vi "TimedTrigger.vi"(8 "error in (no error)":errorcluster, 10 "Time after next UTC Second":T1={"TriggerName"="", "Time after next UTC Second"=0.0, "Trigger Duration"=0.1}, 11 "NiPxi6683H in":refnum<class "NiPxi6683H.lvclass">) -> (0 "error out":errorcluster, 3 "NiPxi6683H out":refnum<class "NiPxi6683H.lvclass">)   [LabVIEW 2014, in "SyncPlugins.lvlib" / "NiPxi6683H.lvclass"]
uses:
  NiPxi6683H.lvclass
  SyncPluginBase/Typedefs/clTimedTrigger.ctl
  NiPxi6683H.lvclass/NiPxi6683H.ctl
  NiPxi6682/NiPxi6682.lvclass/NiPxi6682.ctl
  NiPxi6682/Accessors/Read NiSyncHandle.vi
  NiPxi6682/Accessors/Write NiSyncHandle.vi
  Accessors/Write Triggers.vi
  Accessors/Read Triggers.vi
  <vilib>/Utility/error.llb/Error Cluster From Error Code.vi
  <vilib>/ErrorRing/Error Ring.xnode
  SyncPluginBase/SyncPluginBase.lvclass
panel:
  out "Next PPS 2":timestamp
  out "Next PPS":timestamp
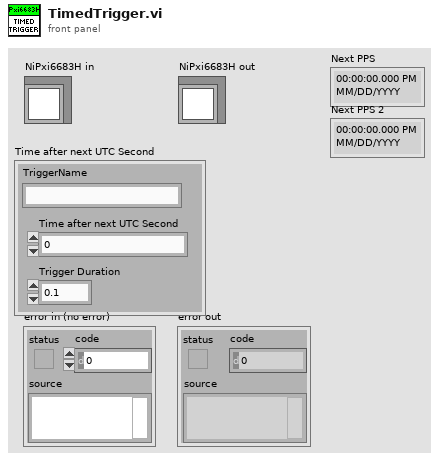
[diagram p1: front panel]
types:
  T1 = typedef "SyncPlugins.lvlib/SyncPluginBase.lvclass/clTimedTrigger.ctl" = cluster{"TriggerName":string, "Time after next UTC Second":dbl, "Trigger Duration":dbl}
  T2 = typedef "SyncPlugins.lvlib/PXI_MultiTrig.lvclass/clTrigger.ctl" = cluster{"Name":string, "DestTerm":string, "SrcTerm":string, "SyncClk":string, "Edge":i32, "Invert?":i32, "Initiated":bool, "Type":string, "TrigTime":bool}
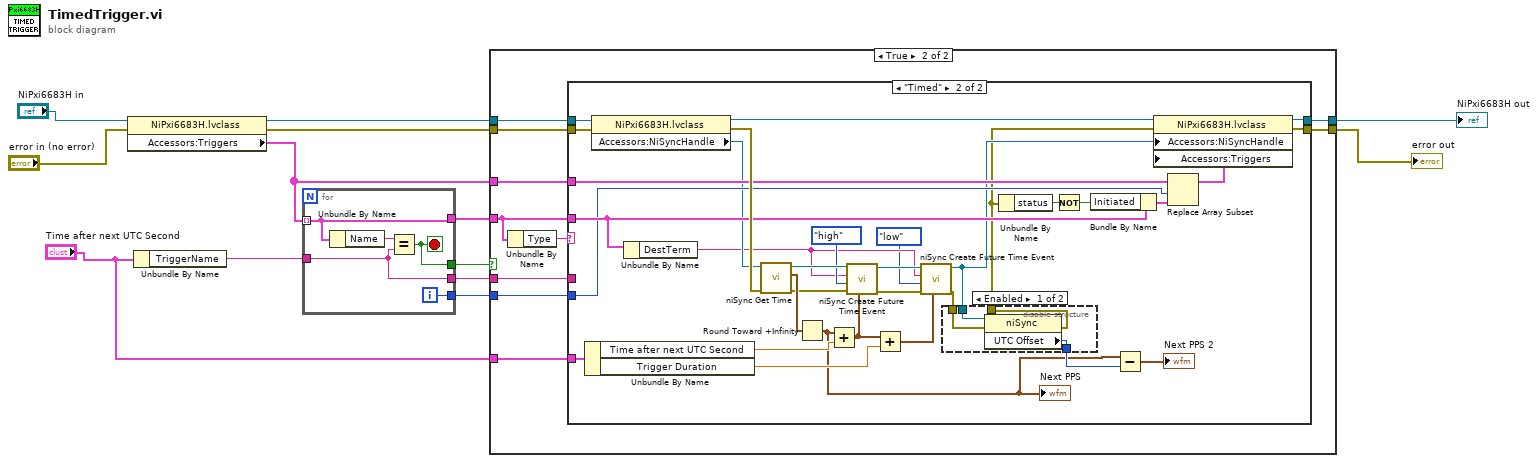
[diagram p0: block diagram]
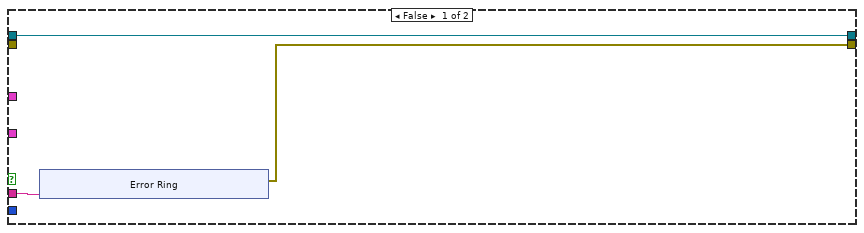
[diagram p2: hidden frame]
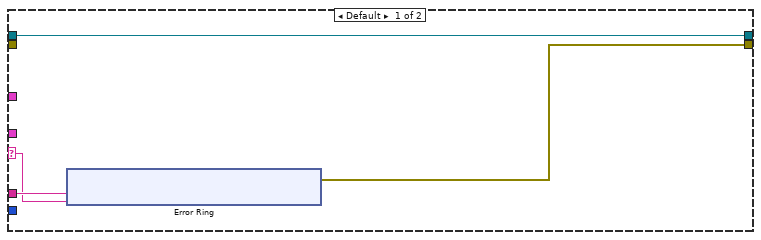
[diagram p3: hidden frame]
diagram:
  n1 = property class="NiPxi6683H.lvclass"(reference="NiPxi6683H in", error in="error in (no error)") -> (reference out=w10:refnum<class "NiPxi6683H.lvclass">, error out=w9:errorcluster, "Accessors:Triggers"=w6:T2[])
  n2 = Unbundle By Name("Time after next UTC Second") -> ("TriggerName"=w13:string)
  n3 = for {
    tunnel: w6 -> [w17] mode=indexing
    tunnel: w13 -> [w15]
    tunnel: [w17] -> w8
    tunnel: [w16] -> w12
    tunnel: [w15] -> w11
    tunnel: [w14] -> w7
    i -> [w14]
    stop <- w16 stop-if-true
    n4 = Unbundle By Name(w17) -> ("Name"=w18:string)
    n5 = Equal?(x=w18, y=w15) -> (x = y?=w16:bool)
  }
  n6 = case shown="True" w12 {
    tunnel: w11 -> [w21 w37]
    tunnel: w10 -> [w20 w32]
    tunnel: w9 -> [_ w30]
    tunnel: [w20 w31] -> w2
    tunnel: [w19 w34] -> w1
    tunnel: w8 -> [_ w33]
    tunnel: w7 -> [_ w36]
    tunnel: w6 -> [_ w35]
    tunnel: "Time after next UTC Second" -> [_ w29]
    frame False {
      n7 = xnode "Error Ring"("parameter 0"=w21) -> ("error out"=w19:errorcluster)
    }
    frame True {
      n8 = Unbundle By Name(w33) -> ("Type"=w38:string)
      n9 = case shown="\"Timed\"" w38 {
        selector: w38 -> [w41 _]
        tunnel: w37 -> [w42 _]
        tunnel: w36 -> [_ w70]
        tunnel: w35 -> [_ w71]
        tunnel: [w40 w76] -> w34
        tunnel: w33 -> [_ w75]
        tunnel: w32 -> [w39 w82]
        tunnel: [w39 w77] -> w31
        tunnel: w30 -> [_ w83]
        tunnel: w29 -> [_ w59]
        frame Default {
          n10 = xnode "Error Ring"("parameter 0"=w42, "parameter 1"=w41) -> ("error out"=w40:errorcluster)
        }
        frame "Timed" {
          n11 = Unbundle By Name(w59) -> ("Time after next UTC Second"=w58:dbl, "Trigger Duration"=w57:dbl)
          n12 = property class="NiPxi6683H.lvclass"(reference=w82, error in=w83) -> (reference out=w78:refnum<class "NiPxi6683H.lvclass">, error out=w81:errorcluster, "Accessors:NiSyncHandle"=w68:refnum<k15>)
          n13 = Unbundle By Name(w75) -> ("DestTerm"=w61:string)
          n14 = call <instrlib>:"niSync Get Time.vi"("error in (no error)"=w81, "instrument handle"=w68) -> ("error out"=w79:errorcluster, "time"=w80:timestamp, "instrument handle out"=w67:refnum<k15>)  [unwired: 5 in]
          n15 = Round Toward +Infinity(x=w80) -> (ceil(x): smallest int >= x=w52:timestamp)
          "Next PPS" <- w52
          n16 = Add(x=w52, y=w58) -> (x+y=w63:timestamp)
          n17 = call <instrlib>:"niSync Create Future Time Event.vi"("time"=w63, "error in (no error)"=w79, "output level"=enum32{"low", "high"}."high", "terminal"=w61, "instrument handle"=w67) -> ("error out"=w65:errorcluster, "instrument handle out"=w64:refnum<k15>)  [unwired: 4 in]
          n18 = Add(x=w63, y=w57) -> (x+y=w62:timestamp)
          n19 = call <instrlib>:"niSync Create Future Time Event.vi"("time"=w62, "error in (no error)"=w65, "output level"=enum32{"low", "high"}."low", "terminal"=w61, "instrument handle"=w64) -> ("error out"=w55:errorcluster, "instrument handle out"=w56:refnum<k15>)  [unwired: 4 in]
          n20 = disable-structure shown="Enabled" {
            disable-tunnel: w56 -> [w87 _]
            disable-tunnel: w55 -> [w86 w88]
            disable-tunnel: [w85 w88] -> w54
            disable-tunnel: [w84 _] -> w53
            frame Enabled {
              n21 = property class="niSync"(reference=w87, error in=w86) -> (error out=w85:errorcluster, "UTC Offset"=w84:i32)  [unwired: 1 out]
            }
            frame Disabled {
            }
          }
          n22 = Unbundle By Name(w54) -> ("status"=w74:bool)
          n23 = Not(x=w74) -> (.not. x?=w73:bool)
          n24 = Bundle By Name(cluster=w75, "Initiated"=w73) -> (w72:T2)
          n25 = Subtract(x=w52, y=w53) -> (x-y=→"Next PPS 2":timestamp)
          n26 = Replace Array Subset(array=w71, new element=w72, index=w70) -> (w69:T2[])
          n27 = property class="NiPxi6683H.lvclass"(reference=w78, error in=w54, "Accessors:NiSyncHandle"=w56, "Accessors:Triggers"=w69) -> (reference out=w77:refnum<class "NiPxi6683H.lvclass">, error out=w76:errorcluster)
        }
      }
    }
  }
  "error out" <- w1
  "NiPxi6683H out" <- w2
